vi "LDA_analogue_start_time_sync_PN.vi"(4 "Correlation peak fit method":enum32{"Max", "Quadratic", "Gaussian"}(ring)=enum."Quadratic", 5 "Pulse high threshold (Volts)":dbl=2.5, 6 "Analogue dt (s)":dbl, 7 "Analogue LDA burst pulse array":dbl[](array[numeric]), 8 "LDA arrival Times":dbl[](array[numeric])) -> (1 "valid bursts checksum status":bool=TRUE, 2 "Absolute LDA times (s)":dbl[](array[numeric]), 3 "LDA start time rel. to Analogue (s)":dbl)   [LabVIEW 2012]
uses:
  <vilib>/Analysis/1siggen.llb/Ramp Pattern by Samples.vi
  <vilib>/Analysis/2dsp.llb/1D Cross Correlation (DBL).vi
  <vilib>/Analysis/polynomials.llb/Polynomial Roots (DBL).vi
  <vilib>/Analysis/polynomials.llb/nth Derivative of Polynomial (DBL).vi
  <vilib>/Analysis/NI_AALPro.lvlib
  <vilib>/Analysis/NI_AALBase.lvlib
panel:
  out "Xcorr LDA timings":cluster{"Ramp Pattern":dbl[], dbl[]}[](graph)
  in  "Pts. either side of peak to use in fit":i32=3
  out "Analogue LDA burst pulse array":cluster{"index (row)":dbl, dbl, "Vout":dbl[]}(graph)
  out "Thresholded LDA burst times (valid only)":cluster{"index (row)":dbl, dbl, "Vout":dbl[]}(graph)
  out "Thresholded LDA arr time checksum":i32
  out "Thresholded LDA burst times (valid + invalid)":cluster{"index (row)":dbl, dbl, "Vout":dbl[]}(graph)
  out "LDA counted pulses (valid + invalid)":i32
  out "LDA arr_t length":i32
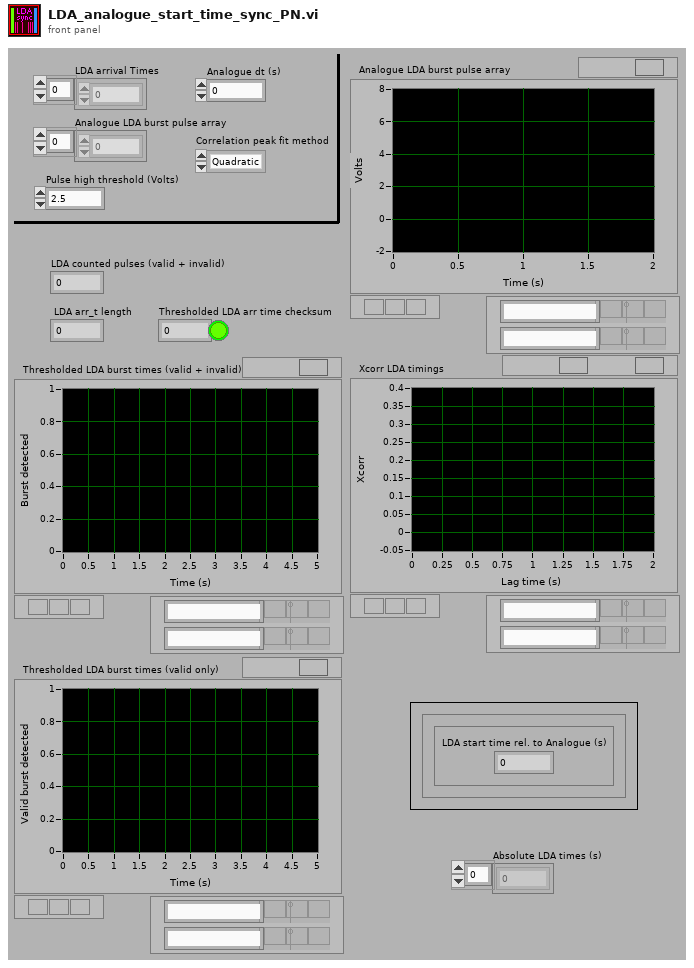
[diagram p1: front panel]
types:
  T1 = cluster{"index (row)":dbl, "Analogue dt (s)":dbl, "Vout":dbl[]}
  T2 = cluster{"index (row)":dbl, "Analogue dt (s)":dbl, "Analogue LDA burst pulse array":dbl[]}
  T3 = cluster{"Ramp Pattern":dbl[], "Best Gaussian Fit":dbl[]}[]
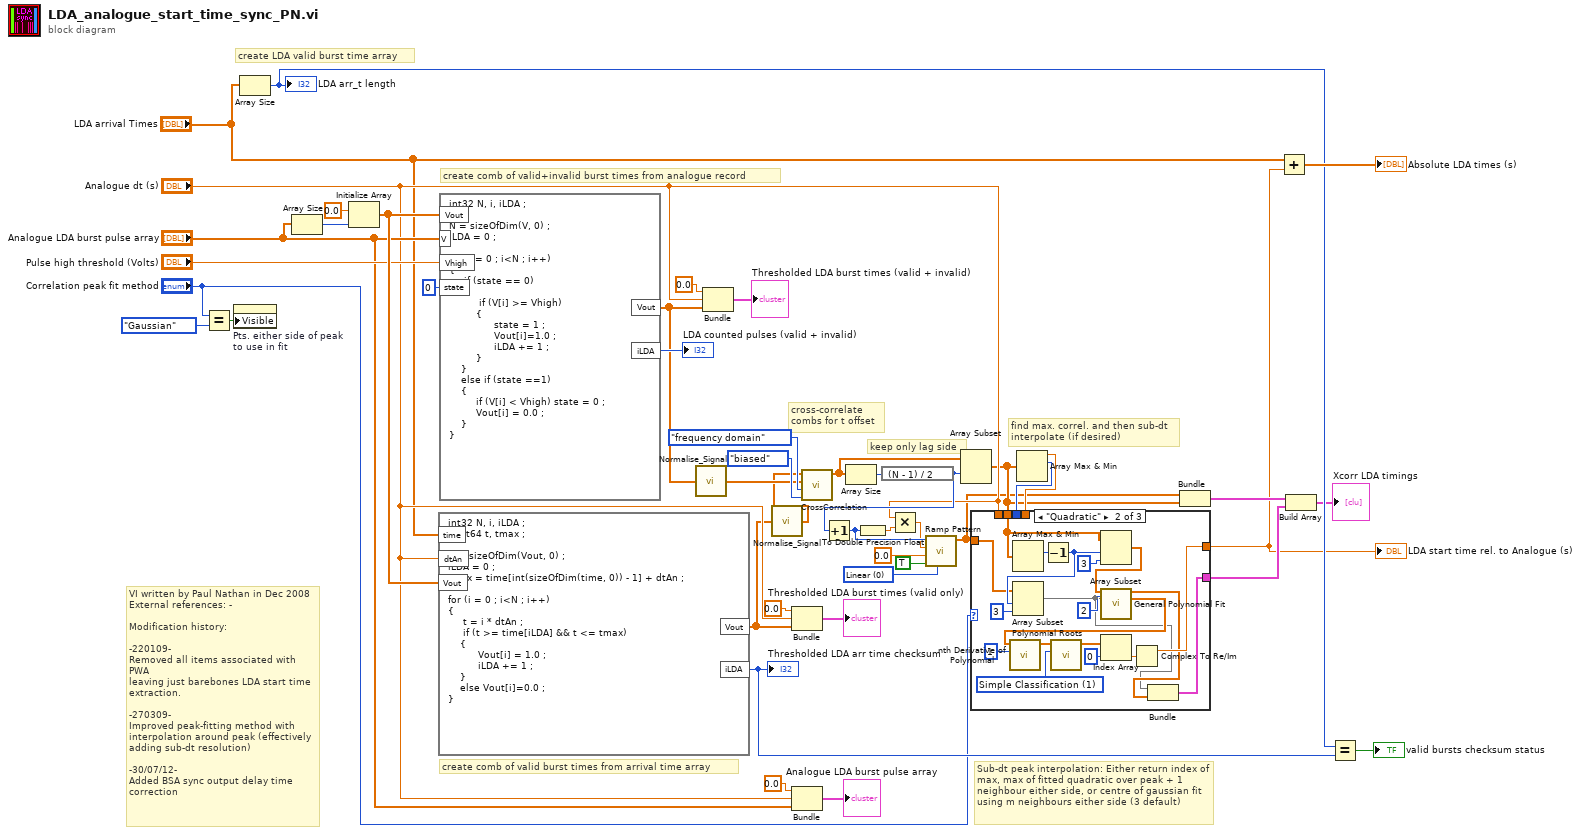
[diagram p0: block diagram]
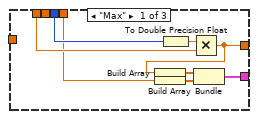
[diagram p2: hidden frame]
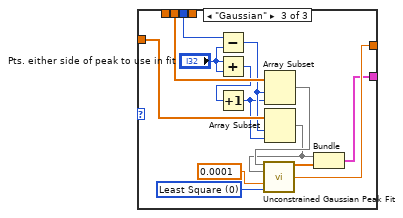
[diagram p3: hidden frame]
diagram:
  w15 = u16 0 items=["Linear", "Logarithmic"] ("type")
  # "find max. correl. and then sub-dt interpolate (if desired)"
  # "Sub-dt peak interpolation: Either return index of max, max of fitted quadratic over peak + 1 neighbour either side, or centre of gaussian fit using m neighbours either side (3 default)"
  # "create LDA valid burst time array"
  # "keep only lag side"
  # "cross-correlate combs for t offset"
  # "VI written by Paul Nathan in Dec 2008\nExternal references: -\n\nModification history:\n\n-220109-\nRemoved all items associated with PWA\nleaving just barebones LDA start time\nextraction.\n\n-270309-\nImproved peak-fitting method with interpolation around peak (effectively adding sub-dt resolution)\n\n-30/07/12-\nAdded BSA sync output delay time correction"
  # "create comb of valid+invalid burst times from analogue record"
  # "create comb of valid burst times from arrival time array"
  n1 = Equal?(x="Correlation peak fit method", y=enum32{"Max", "Quadratic", "Gaussian"}."Gaussian") -> (x = y?=w8:bool)
  n2 = property on="Pts. either side of peak to use in fit" class="DigNum (strict)"("Visible"=w8) -> ()  [unwired: 2 in, 2 out]
  n3 = Array Size(array="LDA arrival Times") -> (size(s)=w30:i32)
  "LDA arr_t length" <- w30
  n4 = Array Size(array="Analogue LDA burst pulse array") -> (size(s)=w35:i32)
  n5 = Initialize Array(0.0 ("element"), w35) -> (w34:dbl[])
  n6 = formula code="int32 N, i, iLDA ;\nfloat64 t, tmax ;\n\nN = sizeOfDim(Vout, 0) ;\niLDA = 0 ;\ntmax = time[int(sizeOfDim(time, 0)) - 1] + dtAn ;\n\nfor (i = 0 ; i<N ; i++)\n{\n     t = i * dtAn ;\n     if (t >= time[iLDA] && t <= tmax) \n    {\n          Vout[i] = 1.0 ;\n          iLDA += 1 ;\n    }\n    else Vout[i]=0.0 ;\n}"("dtAn"="Analogue dt (s)", "time"="LDA arrival Times", "Vout"=w34) -> ("Vout"=w3:dbl[], "iLDA"=w33:i32)
  "Thresholded LDA arr time checksum" <- w33
  n7 = formula code="int32 N, i, iLDA ;\n\nN = sizeOfDim(V, 0) ;\niLDA = 0 ;\n\nfor (i = 0 ; i<N ; i++)\n{\n     if (state == 0) \n    {\n          if (V[i] >= Vhigh)\n         {\n               state = 1 ;\n               Vout[i]=1.0 ;\n               iLDA += 1 ;\n         }\n    }\n    else if (state ==1)\n    {\n         if (V[i] < Vhigh) state = 0 ;\n         Vout[i] = 0.0 ;\n    }\n}"("V"="Analogue LDA burst pulse array", "Vhigh"="Pulse high threshold (Volts)", "state"=u8 0 ("input variable"), "Vout"=w34) -> ("Vout"=w5:dbl[], "iLDA"=→"LDA counted pulses (valid + invalid)":i32)
  n8 = call "Normalise_Signal.vi"("x"=w5) -> ("(x-X)/sigma"=w4:dbl[])  [unwired: 4 in]
  n9 = Bundle("index (row)"=0.0, "Analogue dt (s)"="Analogue dt (s)", "Vout"=w5) -> (→"Thresholded LDA burst times (valid + invalid)":T1)  [unwired: 1 out]
  n10 = call "Normalise_Signal.vi"("x"=w3) -> ("(x-X)/sigma"=w2:dbl[])  [unwired: 4 in]
  n11 = Bundle("index (row)"=0.0, "Analogue dt (s)"="Analogue dt (s)", "Vout"=w3) -> (→"Thresholded LDA burst times (valid only)":T1)  [unwired: 1 out]
  n12 = Bundle("index (row)"=0.0, "Analogue dt (s)"="Analogue dt (s)", "Analogue LDA burst pulse array"="Analogue LDA burst pulse array") -> (→"Analogue LDA burst pulse array":T2)  [unwired: 1 out]
  n13 = call-poly <vilib>:"CrossCorrelation.vi"("normalization"=enum32{"none", "unbiased", "biased"}."biased", "algorithm"=enum32{"direct", "frequency domain"}."frequency domain", "Y"=w4, "X"=w2) -> ("Rxy"=w36:dbl[])  [unwired: 7 out]
  n14 = Array Size(array=w36) -> (size(s)=w37:i32)
  n15 = expression code="(N - 1) / 2"(w37) -> (w17:i32)
  n16 = Increment(x=w17) -> (x+1=w24:i32)
  n17 = To Double Precision Float(number=w24) -> (double precision float=w22:dbl)
  n18 = Multiply(x="Analogue dt (s)", y=w22) -> (x*y=w23:dbl)
  n19 = call-poly <vilib>:"Ramp Pattern.vi"("type"=w15, "exclude end?"=TRUE, "start"=0.0, "end"=w23, "samples"=w24) -> ("Ramp Pattern"=w11:dbl[])  [unwired: 5 in, 1 out]
  n20 = Array Subset(array=w36, index=w17) -> (w12:dbl[])  [unwired: 1 in]
  n21 = Array Max & Min(array=w12) -> (max value=w13:dbl, max index (indices)=w14:i32)  [unwired: 2 out]
  n22 = case shown="\"Quadratic\"" "Correlation peak fit method" {
    tunnel: w12 -> [_ w61 w83]
    tunnel: [w46 w62 w85] -> w6
    tunnel: "Analogue dt (s)" -> [w53 _ _]
    tunnel: [w50 w59 w75] -> w10
    tunnel: w11 -> [_ w55 w80]
    tunnel: w14 -> [w51 _ w82]
    tunnel: w13 -> [w47 _ _]
    frame "Max" {
      n23 = Build Array(w47) -> (w49:dbl[])
      n24 = To Double Precision Float(number=w51) -> (double precision float=w52:dbl)
      n25 = Multiply(x=w52, y=w53) -> (x*y=w46:dbl)
      n26 = Build Array(w46) -> (w48:dbl[])
      n27 = Bundle(w48, w49) -> (w50:cluster{dbl[], dbl[]})  [unwired: 1 out]
    }
    frame "Quadratic" {
      w66 = u16 1 items=["General", "Simple Classification", "Refinement", "Advanced Refinement"] ("option")
      n28 = Array Max & Min(array=w61) -> (max index (indices)=w71:i32)  [unwired: 3 out]
      n29 = Decrement(x=w71) -> (x-1=w56:i32)
      n30 = Array Subset(array=w55, index=w56, length=3) -> (w54:dbl[])
      n31 = Array Subset(array=w61, index=w56, length=3) -> (w70:dbl[])
      n32 = call <vilib>:"General Polynomial Fit.vi"("Y"=w70, "polynomial order"=2, "X"=w54) -> ("Best Polynomial Fit"=w58:dbl[], "Polynomial Coefficients"=w60:dbl[])  [unwired: 9 in, 2 out]
      n33 = call-poly <vilib>:"nth Derivative of Polynomial.vi"("order"=1, "P(x)"=w60) -> ("Nth Derivative of P(x)"=w67:dbl[])  [unwired: 9 out]
      n34 = call-poly <vilib>:"Polynomial Roots.vi"("option"=w66, "P(x)"=w67) -> ("Roots"=w65:cdb[])  [unwired: 9 out]
      n35 = Index Array(array=w65, index=0) -> (element=w63:cdb)
      n36 = Complex To Re/Im(x + iy=w63) -> (x=w62:dbl)  [unwired: 1 out]
      n37 = Bundle(w54, "Best Polynomial Fit"=w58) -> (w59:cluster{dbl[], "Best Polynomial Fit":dbl[]})  [unwired: 1 out]
    }
    frame "Gaussian" {
      w84 = u16 0 items=["Least Square", "Least Absolute Residual", "Bisquare"] ("method")
      n38 = Subtract(x=w82, y="Pts. either side of peak to use in fit") -> (x-y=w79:i32)
      n39 = Add(x="Pts. either side of peak to use in fit", y="Pts. either side of peak to use in fit") -> (x+y=w73:i32)
      n40 = Increment(x=w73) -> (x+1=w74:i32)
      n41 = Array Subset(array=w83, index=w79, length=w74) -> (w78:dbl[])
      n42 = Array Subset(array=w80, index=w79, length=w74) -> (w76:dbl[])
      n43 = call <vilib>:"Unconstrained Gaussian Peak Fit.vi"("Y"=w78, "X"=w76, "tolerance"=0.0001, "method"=w84) -> ("Best Gaussian Fit"=w77:dbl[], "center"=w85:dbl)  [unwired: 6 in, 4 out]
      n44 = Bundle(w76, "Best Gaussian Fit"=w77) -> (w75:cluster{dbl[], "Best Gaussian Fit":dbl[]})  [unwired: 1 out]
    }
  }
  "LDA start time rel. to Analogue (s)" <- w6
  n45 = Bundle("Ramp Pattern"=w11, w12) -> (w18:cluster{"Ramp Pattern":dbl[], dbl[]})  [unwired: 1 out]
  n46 = Add(x="LDA arrival Times", y=w6) -> (x+y=→"Absolute LDA times (s)":dbl[])
  n47 = Build Array(w18, w10) -> (→"Xcorr LDA timings":T3)
  n48 = Equal?(x=w30, y=w33) -> (x = y?=→"valid bursts checksum status":bool)
